vi "UDP Broadcast.vi"(5 "port or service name":u16=61557, 7 "address":u32, 8 "error in (no error)":errorcluster, 9 "timeout ms (25000)":i32=25000, 10 "data in":string, 11 "connection ID":refnum<k16>) -> (0 "error out":errorcluster, 3 "connection ID out":refnum<k16>)   [LabVIEW 2020]
panel:
  out "bytes":i32
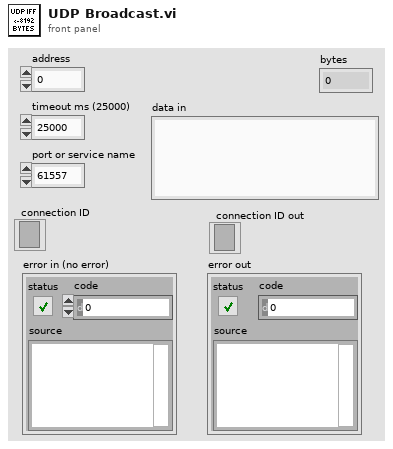
[diagram p1: front panel]
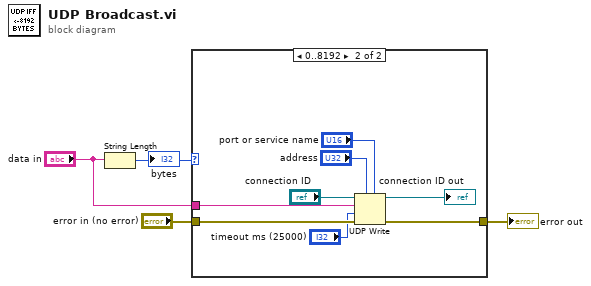
[diagram p0: block diagram]
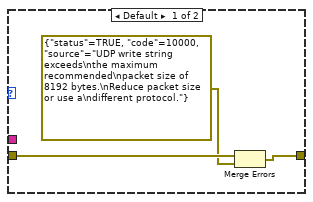
[diagram p2: hidden frame]
diagram:
  n1 = String Length(string="data in") -> (length=w4:i32)
  "bytes" <- w4
  n2 = case shown="0..8192" w4 {
    tunnel: "error in (no error)" -> [w7 w15]
    tunnel: [w6 w14] -> w2
    tunnel: "data in" -> [_ w13]
    frame Default {
      n3 = Merge Errors(w7, errorcluster {"status"=TRUE, "code"=10000, "source"="UDP write string exceeds\nthe maximum recommended\npacket size of 8192 bytes.\nReduce packet size or use a\ndifferent protocol."} ("error constant")) -> (w6:errorcluster)
    }
    frame 0..8192 {
      n4 = UDP Write(address="address", port or service name="port or service name", connection ID="connection ID", data in=w13, 8:w15, 9:"timeout ms (25000)") -> (error out=w14:errorcluster, 3:→"connection ID out":refnum<k16>)
    }
  }
  "error out" <- w2
